vi "subVI_boolean_to_voltage.vi"(9 "Gain":i16, 10 "UNI":i16, 11 "ADC read":bool[](array[boolean])=[TRUE, TRUE, TRUE, FALSE, FALSE, TRUE, TRUE, FALSE, TRUE, FALSE, TRUE, TRUE, FALSE, TRUE, TRUE, FALSE]) -> (3 "V":dbl)   [LabVIEW 2018]
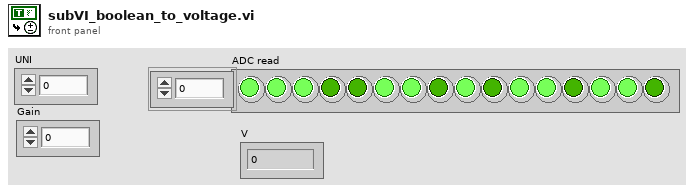
[diagram p1: front panel]
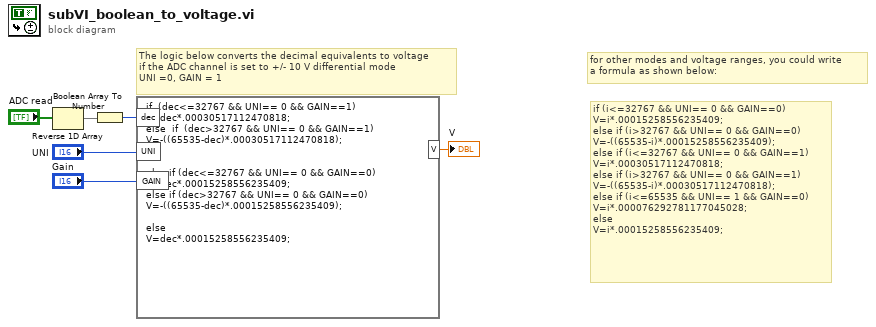
[diagram p0: block diagram]
diagram:
  # "for other modes and voltage ranges, you could write\na formula as shown below:"
  # "The logic below converts the decimal equivalents to voltage\nif the ADC channel is set to +/- 10 V differential mode\nUNI =0, GAIN = 1"
  # "if (i<=32767 && UNI== 0 && GAIN==0)\nV=i*.00015258556235409;\nelse if (i>32767 && UNI== 0 && GAIN==0)\nV=-((65535-i)*.00015258556235409);\nelse if (i<=32767 && UNI== 0 && GAIN==1)\nV=i*.00030517112470818;\nelse if (i>32767 && UNI== 0 && GAIN==1)\nV=-((65535-i)*.00030517112470818);\nelse if (i<=65535 && UNI== 1 && GAIN==0)\nV=i*.000076292781177045028;\nelse\nV=i*.00015258556235409;"
  n1 = Reverse 1D Array(array="ADC read") -> (reversed array=w5:bool[])
  n2 = Boolean Array To Number(Boolean array=w5) -> (number=w4:u16)
  n3 = formula code="if  (dec<=32767 && UNI== 0 && GAIN==1)\nV=dec*.00030517112470818;\nelse  if  (dec>32767 && UNI== 0 && GAIN==1)\nV=-((65535-dec)*.00030517112470818);\n\n\nelse if (dec<=32767 && UNI== 0 && GAIN==0)\nV=dec*.00015258556235409;\nelse if (dec>32767 && UNI== 0 && GAIN==0)\nV=-((65535-dec)*.00015258556235409);\n\nelse\nV=dec*.00015258556235409;"("dec"=w4, "UNI"="UNI", "GAIN"="Gain") -> ("V"=→"V":dbl)
